vi "Thermoreflectance.vi"() -> ()   [LabVIEW 2018]
uses:
  <vilib>/userdefined/High Color/IMAQdx.ctl
  <vilib>/vision/Image Controls.llb/IMAQ Image.ctl
  <vilib>/Platform/TimedLoop/XDataNode/timing_clust.ctl
  <vilib>/Platform/TimedLoop/XDataNode/nitl_modes.ctl
  <vilib>/Platform/TimedLoop/XDataNode/wakeup.ctl
  <vilib>/Utility/file.llb/Write Delimited Spreadsheet (DBL).vi
  <vilib>/Platform/TimedLoop/scheduler/LVUserAPI/_suppVIs/Create_1kHz_TSource.vi
  <vilib>/platform/TimedLoop/XDataNode/XDataNode.xnode
  <vilib>/vision/driver/NI_Vision_Acquisition_Software.lvlib
  <resource>/objmgr/imaqdx.rc
  <instrlib>/Keithley 3390/Keithley 3390.lvlib
  <vilib>/vision/NI_Vision_Development_Module.lvlib
  <vilib>/Platform/TimedLoop/XDataNode/XDNodeRunTimeDep.lvlib
panel:
  in  "Y Resolution":i32=1200
  in  "X Resolution":i32=1600
  out "ImageDiffA":T1[](array[typedef])
  out "ImageColdA":T1[](array[typedef])
  out "ImageHotA":T1[](array[typedef])
  in  "Border Size":i32=1600
  in  "Exposure (us)":u32=1000
  in  "Path":path
  out "Mean":i16[][](array[numeric])
  out "Difference":i16[][](array[numeric])
  out "DiffImagemean":T1
  out "Imagecold":T1
  out "Message":string
  in  "Trigger while adjusting":u16(ring) items=["Disabled", "Show Hot Time", "Show Cold Time"]
  out "Cold DC":dbl
  out "Hot DC":dbl
  out "Period":dbl
  in  "FPS (Hz)":dbl=10.0
  out "S.G.":bool
  out "Signalgen":refnum<visa-resource-name>
  in  "Signal Generator GPIB":refnum<visa-resource-name>="GPIB0::16::INSTR"
  in  "Cold time":dbl=95.0
  in  "Hot time (ms)":dbl=19.0
  out "lightimgBuffer":T1[](array[typedef])
  out "darkimgBuffer":T1[](array[typedef])
  in  "N rep":i32=30
  in  "N image":i32=30
  in  "JUST QUIT":bool
  out "Imagehot":T1
  out "camera":T2
  in  "ADJUSTMENT DONE":bool
  in  "state":enum16{"INIT", "ADJUST", "ACQ", "SAVE", "QUIT"}(ring)
  out "DisplayedImage":T1(plugin-control)
  in  "Camera":T2="cam2"
  # "MEASUREMENT"
  # "TIMING INFO"
  # "Trigger while adjusting initial value"
  # "DEVICES"
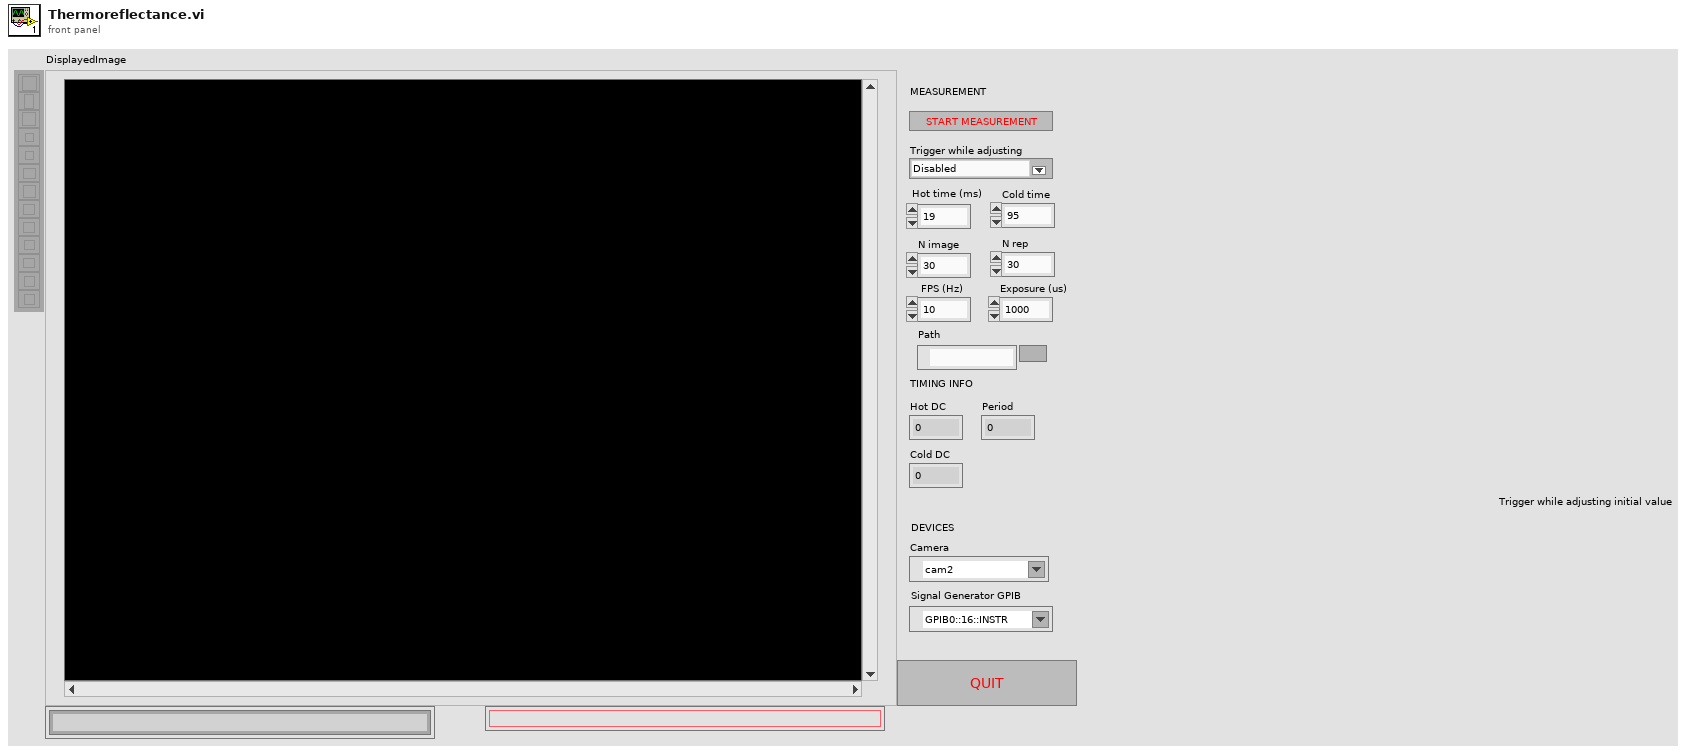
[diagram p1: front panel]
types:
  T1 = typedef "IMAQ Image.ctl" = refnum<image>
  T2 = typedef "IMAQdx.ctl" = refnum<k21>
  T3 = typedef "Image Type" = u32
  T4 = typedef "XDNodeRunTimeDep.lvlib/timing_clust.ctl" = cluster{"Expected End [f-1]":u64, "Actual End [f-1]":u64, "Finished Late? [f-1]":bool, "Expected End [i-1]":u64, "Actual End [i-1]":u64, "Finished Late? [i-1]":bool, "Expected Start [i]":u64, "Actual Start [i]":u64, "Expected Start [f]":u64, "Actual Start [f]":u64, "Source Name":string, "Structure Name":string, "Period":i64, "Deadline":i64, "Offset":i64, "Start":i64, "Priority":i32, "Timeout":i32, "Mode":T5, "Wakeup Reason":T6, "Error":errorcluster, "Source Type":string, "Secondary Source Type":string, "Global End Time":u64, "Global Start Time":u64, "Frame Duration":u64, "Iteration Duration":u64, "Assigned CPU":i32, "I/O Scan Engine Mode":u32}
  T5 = typedef "XDNodeRunTimeDep.lvlib/nitl_modes.ctl" = enum32{"No Change", "Process missed periods, maintain original phase", "Discard missed periods, maintain original phase", "Process missed periods, ignore original phase", "Discard missed periods, ignore original phase"}
  T6 = typedef "XDNodeRunTimeDep.lvlib/wakeup.ctl" = enum32{"Normal", "Aborted", "Asynchronous wakeup", "Timing source error", "Timed loop error", "Timeout"}
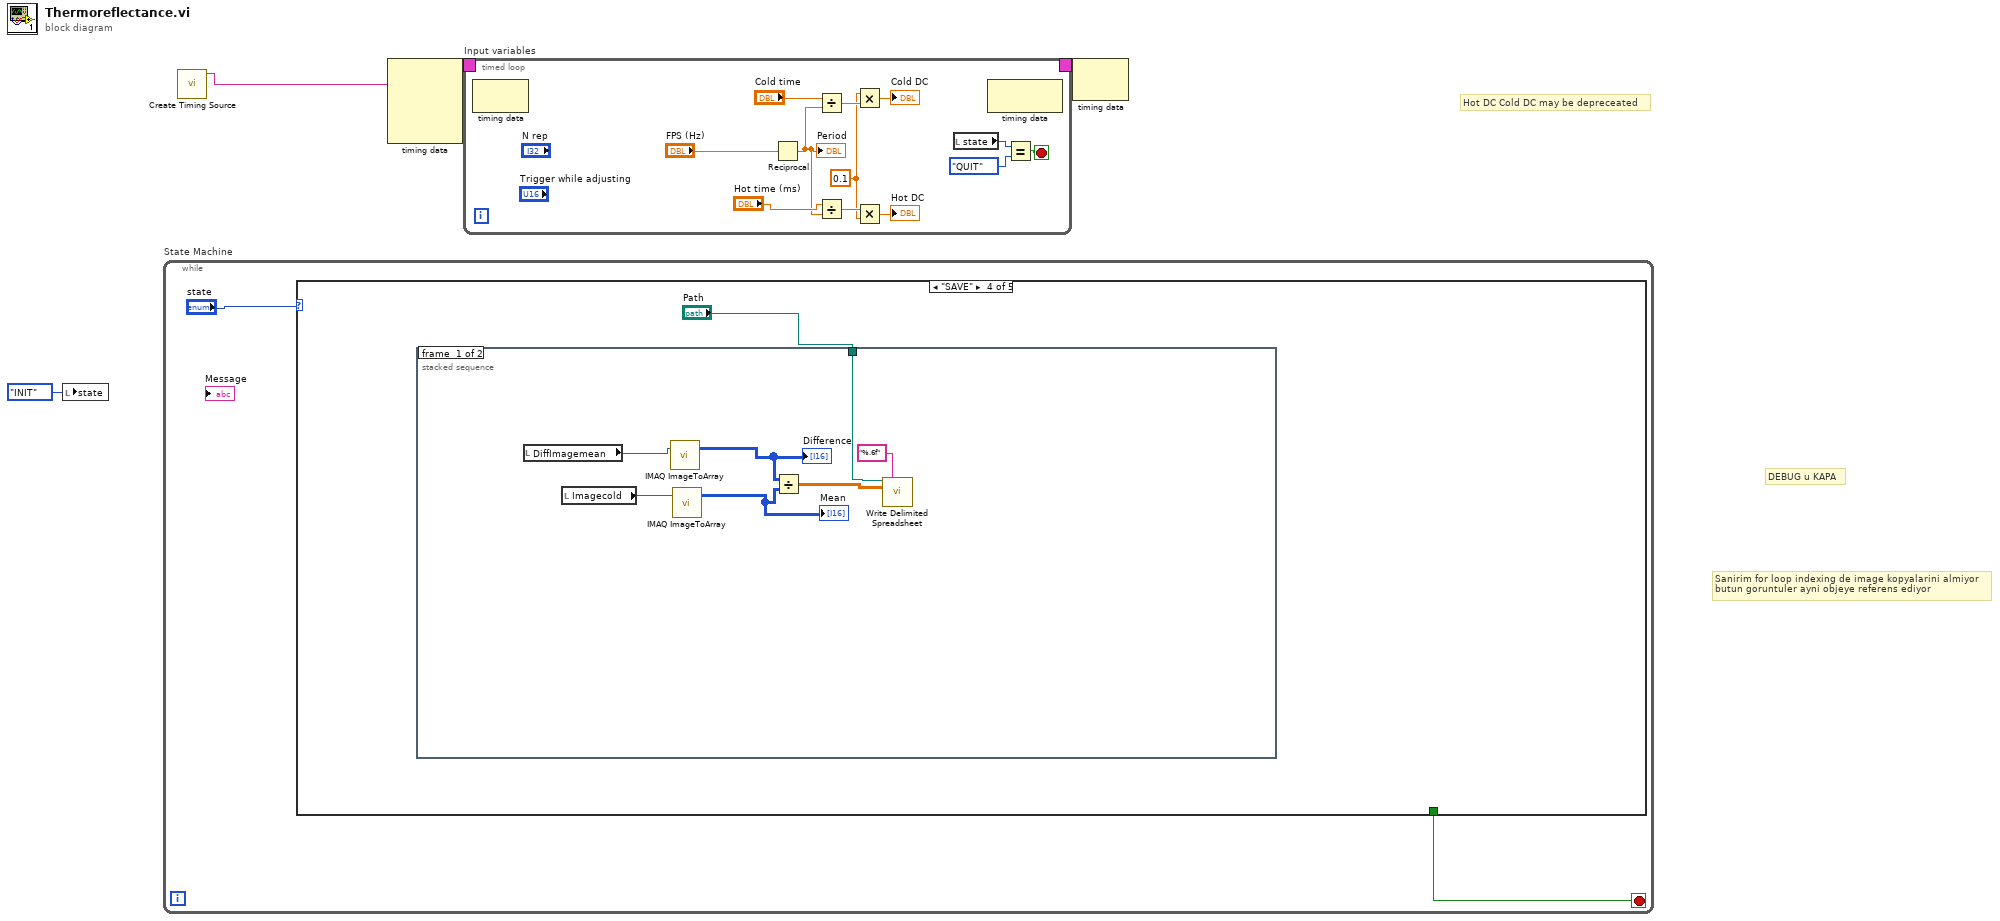
[diagram p0: block diagram]
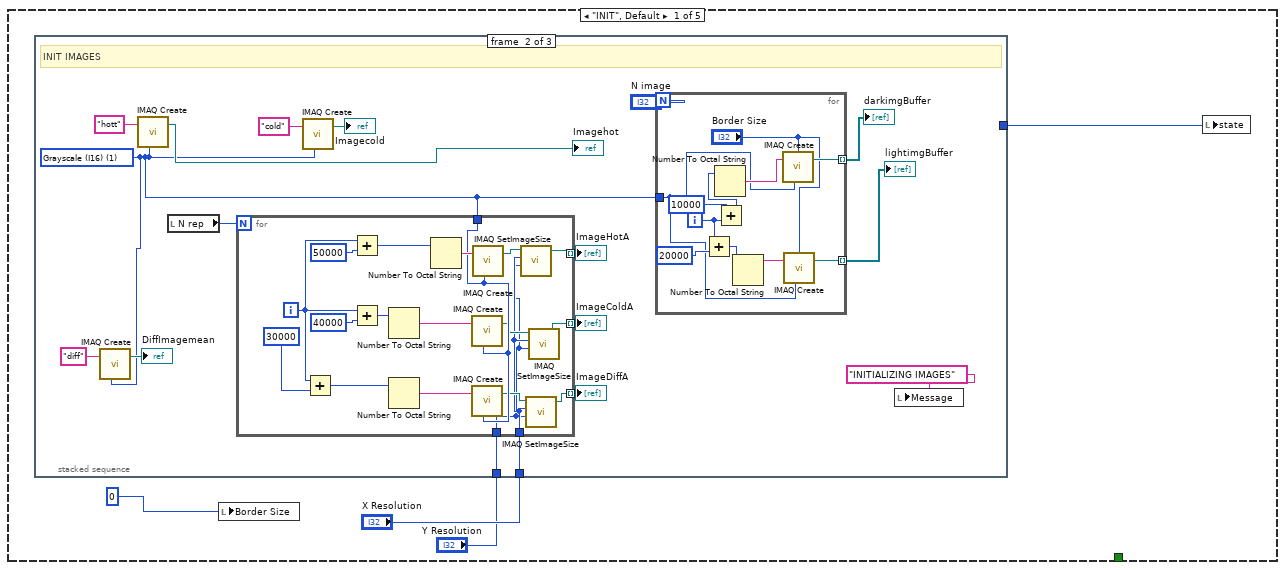
[diagram p2: hidden frame]
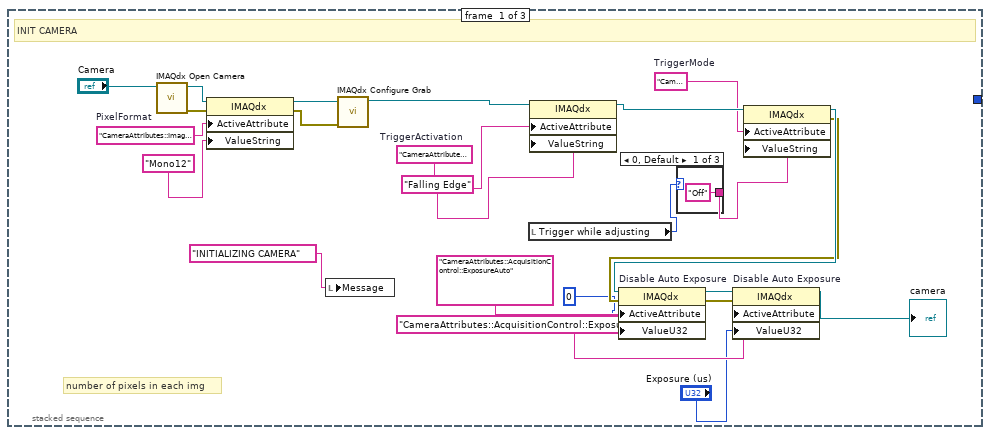
[diagram p3: hidden frame]
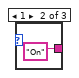
[diagram p4: hidden frame]
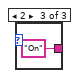
[diagram p5: hidden frame]
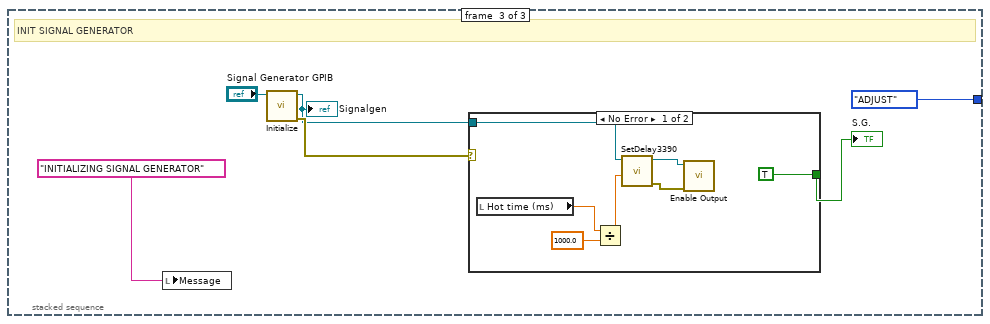
[diagram p6: hidden frame]
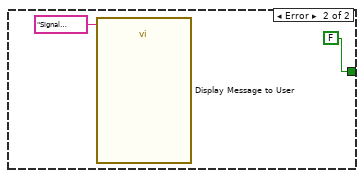
[diagram p7: hidden frame]
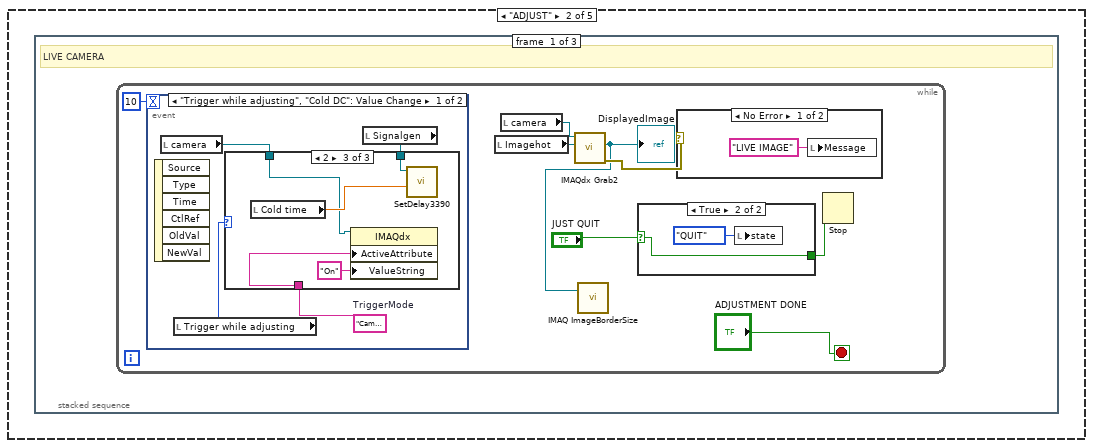
[diagram p8: hidden frame]
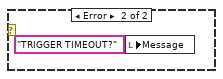
[diagram p9: hidden frame]
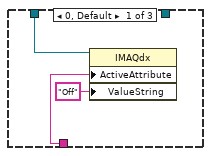
[diagram p10: hidden frame]
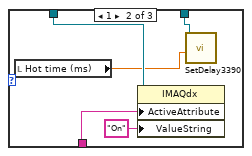
[diagram p11: hidden frame]
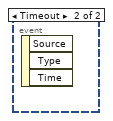
[diagram p12: hidden frame]
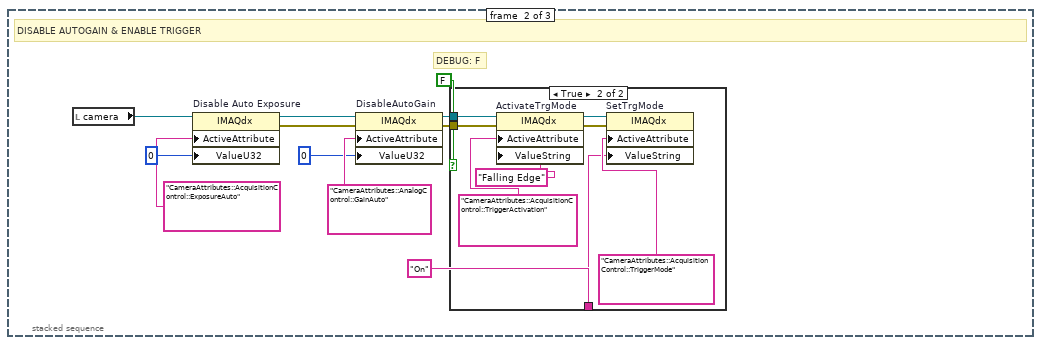
[diagram p14: hidden frame]
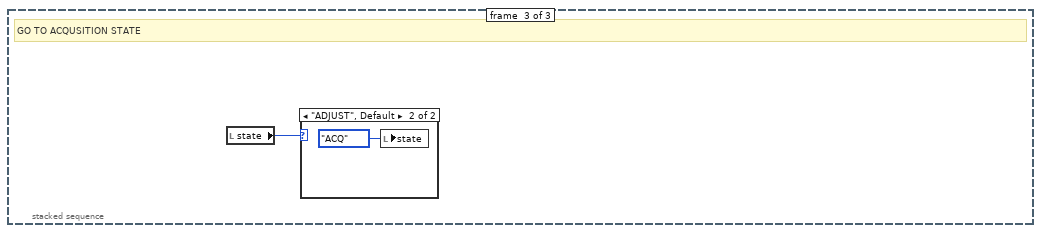
[diagram p16: hidden frame]
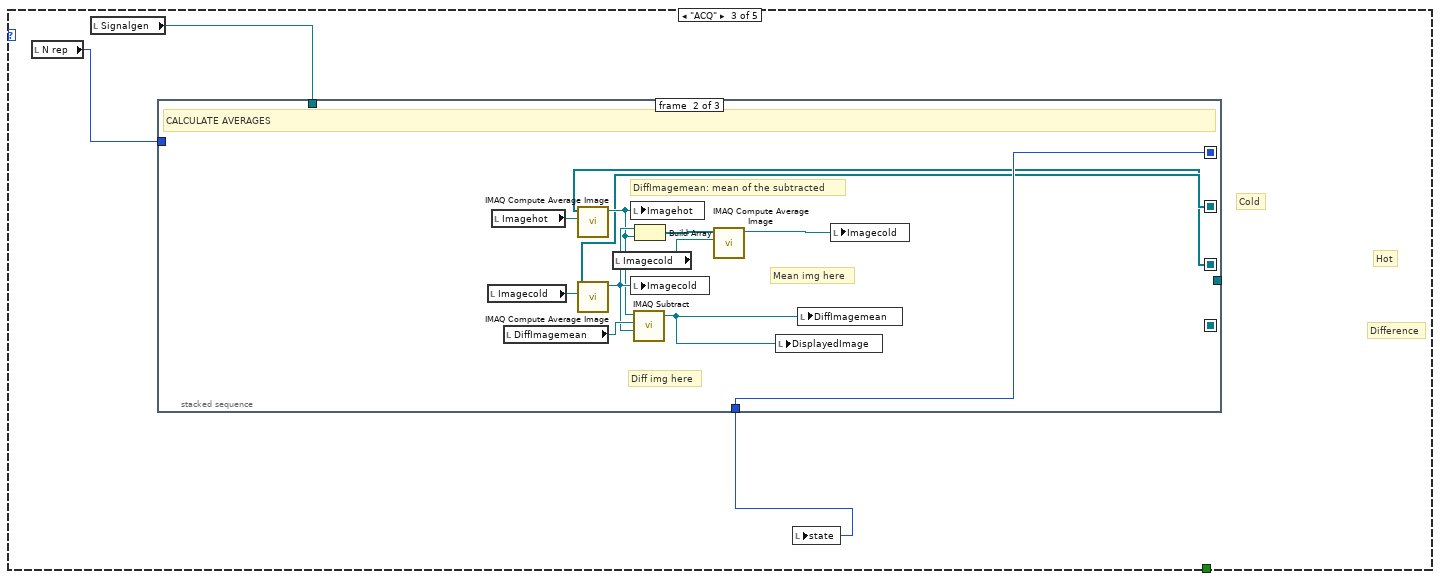
[diagram p18: hidden frame]
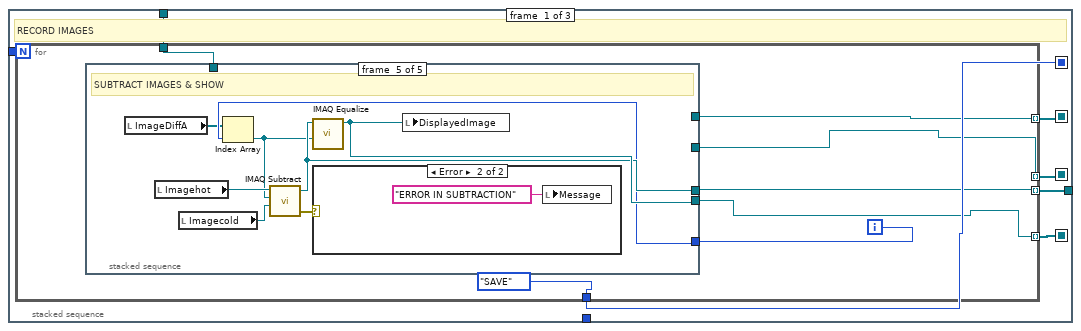
[diagram p19: hidden frame]
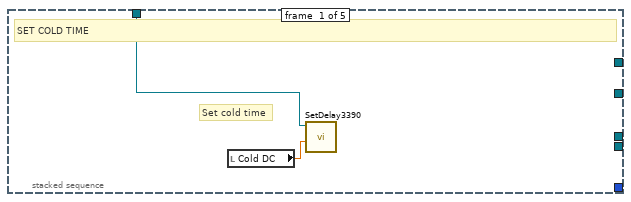
[diagram p20: hidden frame]
diagram:
  # "DEBUG u KAPA"
  # "Sanirim for loop indexing de image kopyalarini almiyor\nbutun goruntuler ayni objeye referens ediyor"
  # "Hot DC Cold DC may be depreceated"
  n1 = local write "state"(enum16{"INIT", "ADJUST", "ACQ", "SAVE", "QUIT"}."INIT" ("state")) -> ()
  n2 = while "State Machine" {
    stop <- w5 stop-if-true
    n3 = case shown="\"SAVE\"" "state" {
      tunnel: [_ _ _ _ TRUE] -> w5
      frame "INIT", Default {
        n4 = stacked-sequence {
          tunnel: [_ _ enum16{"INIT", "ADJUST", "ACQ", "SAVE", "QUIT"}."ADJUST" ("state")] -> w10
          tunnel: "X Resolution" -> [_ w39 _]
          tunnel: "Y Resolution" -> [_ w38 _]
          frame #0 {
            w26 = "CameraAttributes::ImageFormatControl::PixelFormat"  # PixelFormat
            w30 = "CameraAttributes::AcquisitionControl::TriggerMode"  # TriggerMode
            w34 = "CameraAttributes::AcquisitionControl::TriggerActivation"  # TriggerActivation
            # "number of pixels in each img"
            # "INIT CAMERA"
            n5 = call <vilib>:"IMAQdx Open Camera.vi"("Session In"="Camera") -> ("error out"=w23:errorcluster, "Session Out"=w24:T2)  [unwired: 9 in]
            n6 = property class="IMAQdx"(reference=w24, error in=w23, "ActiveAttribute"=w26, "ValueString"="Mono12") -> (reference out=w22:T2, error out=w21:errorcluster)
            n7 = local write "Message"("INITIALIZING CAMERA" ("Message")) -> ()
            n8 = call <vilib>:"IMAQdx Configure Grab.vi"("error in"=w21, "Session In"=w22) -> ("Session Out"=w27:T2)  [unwired: 8 in, 1 out]
            n9 = local read "Trigger while adjusting"() -> (w31:u16)
            n10 = property class="IMAQdx"(reference=w27, "ActiveAttribute"=w34, "ValueString"="Falling Edge") -> (reference out=w32:T2)  [unwired: 1 in, 1 out]
            n11 = case shown="0, Default" w31 {
              tunnel: ["Off" ("ValueString") "On" ("ValueString") "On" ("ValueString")] -> w29
              frame 0, Default {
              }
              frame 1 {
              }
              frame 2 {
              }
            }
            n12 = property class="IMAQdx"(reference=w32, "ActiveAttribute"=w30, "ValueString"=w29) -> (reference out=w19:T2, error out=w18:errorcluster)  [unwired: 1 in]
            n13 = property on="Disable Auto Exposure" class="IMAQdx"(reference=w19, error in=w18, "ActiveAttribute"="CameraAttributes::AcquisitionControl::ExposureAuto", "ValueU32"=u32 0) -> (reference out=w15:T2, error out=w14:errorcluster)
            n14 = property on="Disable Auto Exposure" class="IMAQdx"(reference=w15, error in=w14, "ActiveAttribute"="CameraAttributes::AcquisitionControl::ExposureTime", "ValueU32"="Exposure (us)") -> (reference out=→"camera":T2)  [unwired: 1 out]
          }
          frame #1 {
            w40 = T3 1 items=["Grayscale (U8)", "Grayscale (I16)", "Grayscale (SGL)", "Complex (CSG)", "RGB (U32)", "HSL (U32)", "RGB (U64)", "Grayscale (U16)"] ("Image Type")
            # "INIT IMAGES"
            n15 = call "IMAQ Create"("Image Name"="diff", "Image Type"=w40) -> ("New Image"=→"DiffImagemean":T1)  [unwired: 3 in, 1 out]
            n16 = call "IMAQ Create"("Image Name"="hott", "Image Type"=w40) -> ("New Image"=→"Imagehot":T1)  [unwired: 3 in, 1 out]
            n17 = local read "N rep"() -> (w45:i32)
            n18 = for {
              N: w45 -> [_]
              tunnel: [w61] -> w42 mode=indexing
              tunnel: [w59] -> w43 mode=indexing
              tunnel: [w57] -> w44 mode=indexing
              tunnel: w40 -> [w63]
              tunnel: w39 -> [w56]
              tunnel: w38 -> [w55]
              i -> [w65]
              n19 = Add(x=w65, y=30000 ("x")) -> (x+y=w73:i32)
              n20 = Add(x=w65, y=50000) -> (x+y=w68:i32)
              n21 = Add(x=w65, y=40000) -> (x+y=w72:i32)
              n22 = Number To Octal String(2:w72) -> (0:w69:string)  [unwired: 1 in]
              n23 = Number To Octal String(2:w73) -> (0:w70:string)  [unwired: 1 in]
              n24 = Number To Octal String(2:w68) -> (0:w66:string)  [unwired: 1 in]
              n25 = call "IMAQ Create"("Image Name"=w69, "Image Type"=w63) -> ("New Image"=w60:T1)  [unwired: 3 in, 1 out]
              n26 = call "IMAQ Create"("Image Name"=w70, "Image Type"=w63) -> ("New Image"=w62:T1)  [unwired: 3 in, 1 out]
              n27 = call "IMAQ Create"("Image Name"=w66, "Image Type"=w63) -> ("New Image"=w58:T1)  [unwired: 3 in, 1 out]
              n28 = call "IMAQ SetImageSize"("Y Resolution"=w55, "X Resolution"=w56, "Image"=w58) -> ("Image Out"=w57:T1)  [unwired: 2 in, 1 out]
              n29 = call "IMAQ SetImageSize"("Y Resolution"=w55, "X Resolution"=w56, "Image"=w62) -> ("Image Out"=w61:T1)  [unwired: 2 in, 1 out]
              n30 = call "IMAQ SetImageSize"("Y Resolution"=w55, "X Resolution"=w56, "Image"=w60) -> ("Image Out"=w59:T1)  [unwired: 2 in, 1 out]
            }
            "ImageHotA" <- w44
            "ImageColdA" <- w43
            "ImageDiffA" <- w42
            n31 = call "IMAQ Create"("Image Name"="cold", "Image Type"=w40) -> ("New Image"=→"Imagecold":T1)  [unwired: 3 in, 1 out]
            n32 = for {
              N: "N image" -> [_]
              tunnel: w40 -> [w74]
              tunnel: [w81] -> w47 mode=indexing
              tunnel: [w75] -> w46 mode=indexing
              i -> [w78]
              n33 = Add(x=w78, y=20000) -> (x+y=w77:i32)
              n34 = Add(x=10000, y=w78) -> (x+y=w84:i32)
              n35 = Number To Octal String(2:w84) -> (0:w83:string)  [unwired: 1 in]
              n36 = Number To Octal String(2:w77) -> (0:w79:string)  [unwired: 1 in]
              n37 = call "IMAQ Create"("Border Size"="Border Size", "Image Name"=w83, "Image Type"=w74) -> ("New Image"=w81:T1)  [unwired: 2 in, 1 out]
              n38 = call "IMAQ Create"("Border Size"="Border Size", "Image Name"=w79, "Image Type"=w74) -> ("New Image"=w75:T1)  [unwired: 2 in, 1 out]
            }
            "darkimgBuffer" <- w47
            "lightimgBuffer" <- w46
            n39 = local write "Message"("INITIALIZING IMAGES" ("Message")) -> ()
          }
          frame #2 {
            # "INIT SIGNAL GENERATOR"
            n40 = local write "Message"("INITIALIZING SIGNAL GENERATOR" ("String")) -> ()
            n41 = call <instrlib>:"Initialize.vi"("VISA resource name"="Signal Generator GPIB") -> ("error out"=w89:errorcluster, "VISA resource name out"=w87:refnum<visa-resource-name>)  [unwired: 9 in]
            "Signalgen" <- w87
            n42 = case shown="No Error" w89 {
              tunnel: [TRUE ("S.G.") FALSE ("S.G.")] -> w88
              tunnel: w87 -> [w96 _]
              frame No Error {
                n43 = local read "Hot time (ms)"() -> (w93:dbl)
                n44 = Divide(x=w93, y=1000.0) -> (x/y=w92:dbl)
                n45 = call "SetDelay3390.vi"("ms Delay (pulse width)"=w92, "VISA Refnum in"=w96) -> ("error out"=w94:errorcluster, "VISA resource name out"=w95:refnum<visa-resource-name>)  [unwired: 8 in]
                n46 = call <instrlib>:"Enable Output.vi"("error in (no error)"=w94, "VISA resource name"=w95) -> ()  [unwired: 8 in, 2 out]
              }
              frame Error {
                n47 = call "Display Message to User"("Message"="Signal generator not connected") -> ()  [unwired: 9 in, 2 out]
              }
            }
            "S.G." <- w88
          }
        }
        n48 = local write "Border Size"(0) -> ()
        n49 = local write "state"(w10) -> ()
      }
      frame "ADJUST" {
        n50 = stacked-sequence {
          frame #0 {
            # "LIVE CAMERA"
            n51 = while {
              stop <- "ADJUSTMENT DONE" stop-if-true
              n52 = event shown="[0] \"Trigger while adjusting\", \"Cold DC\": Value Change" {
                selector: _ -> [_ _]
                dyn-events: _ -> [_ _]
                timeout: 10 -> [_ _]
                event "Trigger while adjusting", "Cold DC": Value Change {
                  w112 = "CameraAttributes::AcquisitionControl::TriggerMode"  # TriggerMode
                  n53 = event-data() -> ()  [unwired: 1 in, 6 out]
                  n54 = local read "camera"() -> (w113:T2)
                  n55 = local read "Trigger while adjusting"() -> (w110:u16)
                  n56 = local read "Signalgen"() -> (w111:refnum<visa-resource-name>)
                  n57 = case shown="2" w110 {
                    tunnel: w113 -> [w115 w120 w124]
                    tunnel: w112 -> [w114 w119 w123]
                    tunnel: w111 -> [_ w118 w122]
                    frame 0, Default {
                      n58 = property class="IMAQdx"(reference=w115, "ActiveAttribute"=w114, "ValueString"="Off") -> ()  [unwired: 1 in, 2 out]
                    }
                    frame 1 {
                      n59 = local read "Hot time (ms)"() -> (w117:dbl)
                      n60 = property class="IMAQdx"(reference=w120, "ActiveAttribute"=w119, "ValueString"="On") -> ()  [unwired: 1 in, 2 out]
                      n61 = call "SetDelay3390.vi"("ms Delay (pulse width)"=w117, "VISA Refnum in"=w118) -> ()  [unwired: 8 in, 2 out]
                    }
                    frame 2 {
                      n62 = local read "Cold time"() -> (w126:dbl)
                      n63 = property class="IMAQdx"(reference=w124, "ActiveAttribute"=w123, "ValueString"="On") -> ()  [unwired: 1 in, 2 out]
                      n64 = call "SetDelay3390.vi"("ms Delay (pulse width)"=w126, "VISA Refnum in"=w122) -> ()  [unwired: 8 in, 2 out]
                    }
                  }
                }
                event Timeout {
                  n65 = event-data() -> ()  [unwired: 1 in, 3 out]
                }
              }
              n66 = local read "Imagehot"() -> (w106:T1)
              n67 = local read "camera"() -> (w107:T2)
              n68 = call <vilib>:"IMAQdx Grab2.vi"("Image In"=w106, "Session In"=w107) -> ("error out"=w101:errorcluster, "Image Out"=w100:T1)  [unwired: 6 in, 2 out]
              "DisplayedImage" <- w100
              n69 = call "IMAQ ImageBorderSize"("Image"=w100) -> ()  [unwired: 3 in, 3 out]
              n70 = case shown="True" "JUST QUIT" {
                selector: "JUST QUIT" -> [_ w127]
                tunnel: [_ w127] -> w103
                frame False {
                }
                frame True {
                  n71 = local write "state"(enum16{"INIT", "ADJUST", "ACQ", "SAVE", "QUIT"}."QUIT" ("state")) -> ()
                }
              }
              n72 = case shown="No Error" w101 {
                frame No Error {
                  n73 = local write "Message"("LIVE IMAGE" ("Message")) -> ()
                }
                frame Error {
                  n74 = local write "Message"("TRIGGER TIMEOUT?" ("String")) -> ()
                }
              }
              n75 = Stop(stop? (T)=w103) -> ()
            }
          }
          frame #1 {
            # "DEBUG: F"
            # "DISABLE AUTOGAIN & ENABLE TRIGGER"
            n76 = local read "camera"() -> (w135:T2)
            n77 = property on="Disable Auto Exposure" class="IMAQdx"(reference=w135, "ActiveAttribute"="CameraAttributes::AcquisitionControl::ExposureAuto", "ValueU32"=u32 0) -> (reference out=w134:T2, error out=w133:errorcluster)  [unwired: 1 in]
            n78 = property on="DisableAutoGain" class="IMAQdx"(reference=w134, error in=w133, "ActiveAttribute"="CameraAttributes::AnalogControl::GainAuto", "ValueU32"=u32 0) -> (reference out=w132:T2, error out=w131:errorcluster)
            n79 = case shown="True" FALSE ("Debug") {
              tunnel: w132 -> [_ w147]
              tunnel: w131 -> [_ w146]
              tunnel: "On" ("ValueString") -> [_ w140]
              frame False {
              }
              frame True {
                n80 = property on="ActivateTrgMode" class="IMAQdx"(reference=w147, error in=w146, "ActiveAttribute"="CameraAttributes::AcquisitionControl::TriggerActivation", "ValueString"="Falling Edge") -> (reference out=w145:T2, error out=w144:errorcluster)
                n81 = property on="SetTrgMode" class="IMAQdx"(reference=w145, error in=w144, "ActiveAttribute"="CameraAttributes::AcquisitionControl::TriggerMode", "ValueString"=w140) -> ()  [unwired: 2 out]
              }
            }
          }
          frame #2 {
            # "GO TO ACQUSITION STATE"
            n82 = local read "state"() -> (w148:enum16{"INIT", "ADJUST", "ACQ", "SAVE", "QUIT"})
            n83 = case shown="\"ADJUST\", Default" w148 {
              frame "QUIT" {
              }
              frame "ADJUST", Default {
                n84 = local write "state"(enum16{"INIT", "ADJUST", "ACQ", "SAVE", "QUIT"}."ACQ" ("state")) -> ()
              }
            }
          }
        }
      }
      frame "ACQ" {
        # "Difference"
        # "Hot"
        # "Cold"
        n85 = local read "N rep"() -> (w151:i32)
        n86 = local read "Signalgen"() -> (w152:refnum<visa-resource-name>)
        n87 = stacked-sequence {
          seq-local: [w155 _ _] -> [_ w211 _]
          seq-local: [w157 _ _] -> [_ w205 _]
          seq-local: [w156 _ _] -> [_ w204 _]
          seq-local: [w154 _ _] -> [_ _ _]
          tunnel: w152 -> [w159 _ _]
          tunnel: w151 -> [w158 _ _]
          tunnel: [_ w211 _] -> w150
          tunnel: [w153 _ _] -> _
          frame #0 {
            # "RECORD IMAGES"
            n88 = for {
              N: w158 -> [_]
              tunnel: w159 -> [w166]
              tunnel: [w165] -> w157 mode=indexing
              tunnel: [w164] -> w156 mode=indexing
              tunnel: [enum16{"INIT", "ADJUST", "ACQ", "SAVE", "QUIT"}."SAVE" ("state")] -> w155
              tunnel: [w160] -> w154 mode=indexing
              tunnel: [w161] -> w153 mode=indexing
              i -> [w162]
              n89 = stacked-sequence {
                tunnel: w166 -> [w168 _ w181 _ _]
                tunnel: [_ w169 _ _ _] -> w165
                tunnel: [_ _ _ w185 _] -> w164
                tunnel: [_ _ _ _ w197] -> w160
                tunnel: w162 -> [_ w170 _ w183 w195]
                tunnel: [_ _ _ _ w196] -> w161
                frame #0 {
                  # "Set cold time"
                  # "SET COLD TIME"
                  n90 = local read "Cold DC"() -> (w167:dbl)
                  n91 = call "SetDelay3390.vi"("ms Delay (pulse width)"=w167, "VISA Refnum in"=w168) -> ()  [unwired: 8 in, 2 out]
                }
                frame #1 {
                  (unwired) "ack started" ("message")
                  # "Measure image"
                  # "RECORD COLD IMAGE"
                  n92 = local read "darkimgBuffer"() -> (w177:T1[])
                  n93 = local read "camera"() -> (w176:T2)
                  n94 = call <vilib>:"IMAQdx Sequence2.vi"("Timeout (ms)"=10000, "Images In"=w177, "Session In"=w176) -> ("error out"=w174:errorcluster, "Images Out"=w173:T1[])  [unwired: 6 in, 1 out]
                  n95 = local write "darkimgBuffer"(w173) -> ()
                  n96 = case shown="Error" w174 {
                    frame No Error {
                      n97 = local write "Message"("ACQUIRING IMAGES" ("Message")) -> ()
                    }
                    frame Error {
                      n98 = local write "Message"("ACQ TIMEOUT " ("Message")) -> ()
                    }
                  }
                  n99 = local read "ImageColdA"() -> (w172:T1[])
                  n100 = Index Array(array=w172, index=w170) -> (element=w171:T1)
                  n101 = call "IMAQ Compute Average Image"("Image Dst"=w171, "Images"=w173) -> ("Image Dst Out"=w169:T1)  [unwired: 8 in, 1 out]
                }
                frame #2 {
                  # "Set hot time"
                  # "SET HOT TIME"
                  n102 = local read "Hot DC"() -> (w180:dbl)
                  n103 = call "SetDelay3390.vi"("ms Delay (pulse width)"=w180, "VISA Refnum in"=w181) -> ()  [unwired: 8 in, 2 out]
                }
                frame #3 {
                  (unwired) "avk started" ("message")
                  # "Measure image"
                  # "RECORD HOT IMAGE"
                  n104 = local read "lightimgBuffer"() -> (w190:T1[])
                  n105 = local read "camera"() -> (w189:T2)
                  n106 = call <vilib>:"IMAQdx Sequence2.vi"("Timeout (ms)"=10000, "Images In"=w190, "Session In"=w189) -> ("error out"=w187:errorcluster, "Images Out"=w186:T1[])  [unwired: 6 in, 1 out]
                  n107 = local write "lightimgBuffer"(w186) -> ()
                  n108 = case shown="No Error" w187 {
                    frame No Error {
                      n109 = local write "Message"("ACQUIRING IMAGES" ("Message")) -> ()
                    }
                    frame Error {
                      n110 = local write "Message"("ACQ TIMEOUT " ("Message")) -> ()
                    }
                  }
                  n111 = local read "ImageHotA"() -> (w184:T1[])
                  n112 = Index Array(array=w184, index=w183) -> (element=w182:T1)
                  n113 = call "IMAQ Compute Average Image"("Image Dst"=w182, "Images"=w186) -> ("Image Dst Out"=w185:T1)  [unwired: 8 in, 1 out]
                  n114 = local write "Imagehot"(w185) -> ()
                }
                frame #4 {
                  # "SUBTRACT IMAGES & SHOW"
                  n115 = local read "ImageDiffA"() -> (w194:T1[])
                  n116 = local read "Imagehot"() -> (w200:T1)
                  n117 = local read "Imagecold"() -> (w199:T1)
                  n118 = Index Array(array=w194, index=w195) -> (element=w193:T1)
                  n119 = call "IMAQ Subtract"("Image Src A"=w200, "Image Dst"=w193, "Image Src B"=w199) -> ("Image Dst Out"=w196:T1, "error out"=w198:errorcluster)  [unwired: 4 in]
                  n120 = call "IMAQ Equalize"("Image Dst"=w193, "Image Src"=w196) -> ("Image Dst Out"=w197:T1)  [unwired: 8 in, 1 out]
                  n121 = case shown="Error" w198 {
                    frame No Error {
                      n122 = local write "Message"("SUBTRACTING IMAGES" ("Message")) -> ()
                    }
                    frame Error {
                      n123 = local write "Message"("ERROR IN SUBTRACTION" ("Message")) -> ()
                    }
                  }
                  n124 = local write "DisplayedImage"(w197) -> ()
                }
              }
            }
          }
          frame #1 {
            # "Diff img here"
            # "Mean img here"
            # "DiffImagemean: mean of the subtracted"
            # "CALCULATE AVERAGES"
            n125 = local read "Imagecold"() -> (w212:T1)
            n126 = local read "Imagehot"() -> (w213:T1)
            n127 = local read "DiffImagemean"() -> (w214:T1)
            n128 = call "IMAQ Compute Average Image"("Image Dst"=w213, "Images"=w204) -> ("Image Dst Out"=w209:T1)  [unwired: 8 in, 1 out]
            n129 = call "IMAQ Compute Average Image"("Image Dst"=w212, "Images"=w205) -> ("Image Dst Out"=w210:T1)  [unwired: 8 in, 1 out]
            n130 = local read "Imagecold"() -> (w207:T1)
            n131 = local write "Imagehot"(w209) -> ()
            n132 = local write "Imagecold"(w210) -> ()
            n133 = call "IMAQ Subtract"("Image Src A"=w209, "Image Dst"=w214, "Image Src B"=w210) -> ("Image Dst Out"=w203:T1)  [unwired: 4 in, 1 out]
            n134 = Build Array(w210, w209) -> (w208:T1[])
            n135 = call "IMAQ Compute Average Image"("Image Dst"=w207, "Images"=w208) -> ("Image Dst Out"=w206:T1)  [unwired: 8 in, 1 out]
            n136 = local write "DisplayedImage"(w203) -> ()
            n137 = local write "DiffImagemean"(w203) -> ()
            n138 = local write "Imagecold"(w206) -> ()
          }
          frame #2 {
            # "GO TO SAVE"
            n139 = local write "state"(enum16{"INIT", "ADJUST", "ACQ", "SAVE", "QUIT"}."SAVE" ("state")) -> ()
          }
        }
        n140 = local write "state"(w150) -> ()
      }
      frame "SAVE" {
        n141 = stacked-sequence {
          tunnel: "Path" -> [w223 _]
          frame #0 {
            n142 = local read "DiffImagemean"() -> (w222:T1)
            n143 = local read "Imagecold"() -> (w221:T1)
            n144 = call "IMAQ ImageToArray"("Image"=w222) -> ("Image Pixels (I16)"=w220:i16[][])  [unwired: 3 in, 4 out]
            "Difference" <- w220
            n145 = call "IMAQ ImageToArray"("Image"=w221) -> ("Image Pixels (I16)"=w219:i16[][])  [unwired: 3 in, 4 out]
            "Mean" <- w219
            n146 = Divide(x=w220, y=w219) -> (x/y=w218:dbl[][])
            n147 = call-poly <vilib>:"Write Delimited Spreadsheet.vi"("file path (dialog if empty)"=w223, "format (%.3f)"="%.6f", "2D data"=w218) -> ()  [unwired: 11 in, 2 out]
          }
          frame #1 {
            n148 = local write "state"(enum16{"INIT", "ADJUST", "ACQ", "SAVE", "QUIT"}."QUIT" ("state")) -> ()
          }
        }
      }
      frame "QUIT" {
        n149 = local read "camera"() -> (w226:T2)
        n150 = flat-sequence {
          tunnel: w226 -> [w231]
          tunnel: [w231] -> w225
          tunnel: [w233] -> w229
          tunnel: [w234] -> w228
          tunnel: w225 -> [w232]
          tunnel: w229 -> [w237]
          tunnel: w228 -> [w236]
          frame #0 {
            n151 = local write "Message"("QUITTING" ("Message")) -> ()
          }
          frame #1 {
            n152 = call <vilib>:"IMAQdx Stop Acquisition.vi"("Session In"=w232) -> ("error out"=w233:errorcluster, "Session Out"=w234:T2)  [unwired: 9 in]
            n153 = Wait (ms)(milliseconds to wait=u32 1000) -> ()  [unwired: 1 out]
          }
          frame #2 {
            n154 = call <vilib>:"IMAQdx Close Camera.vi"("error in"=w237, "Session In"=w236) -> ()  [unwired: 9 in, 1 out]
          }
        }
      }
    }
  }
  n155 = call-poly <vilib>:"Create Timing Source.vi"() -> ("name (out)"=w1:string)  [unwired: 10 in, 1 out]
  n156 = node-c288(w1) -> (w3:T4)  [unwired: 3 in]
  n157 = timed-loop "Input variables" {
    timing: w3 -> [_]
    timing-out: [_] -> w2
    stop <- w241 stop-if-true
    w244 = 0.1 ("y")
    n158 = node-c288() -> ()  [unwired: 1 in, 1 out]
    n159 = Reciprocal(x="FPS (Hz)") -> (1/x=w238:dbl)
    "Period" <- w238
    n160 = Divide(x="Cold time", y=w238) -> (x/y=w246:dbl)
    n161 = Divide(x="Hot time (ms)", y=w238) -> (x/y=w248:dbl)
    n162 = Multiply(x=w244, y=w246) -> (x*y=→"Cold DC":dbl)
    n163 = Multiply(x=w248, y=w244) -> (x*y=→"Hot DC":dbl)
    n164 = local read "state"() -> (w243:enum16{"INIT", "ADJUST", "ACQ", "SAVE", "QUIT"})
    n165 = node-c288() -> ()  [unwired: 1 in, 1 out]
    n166 = Equal?(x=w243, y=enum16{"INIT", "ADJUST", "ACQ", "SAVE", "QUIT"}."QUIT" ("state")) -> (x = y?=w241:bool)
  }
  n167 = node-c288(w2) -> ()  [unwired: 1 out]
